vi "ADCP_write_data_packet_to_serial_port.vi"(8 "error in (no error)":errorcluster, 9 "Frame Index":i32=-1, 10 "Frame name":string, 11 "ADCP in":refnum<class "ADCP.lvclass">) -> (0 "error out":errorcluster, 3 "ADCP out":refnum<class "ADCP.lvclass">)   [LabVIEW 2017, in "ADCP.lvclass"]
uses:
  ADCP.lvclass
  ADCP.lvclass/ADCP.ctl
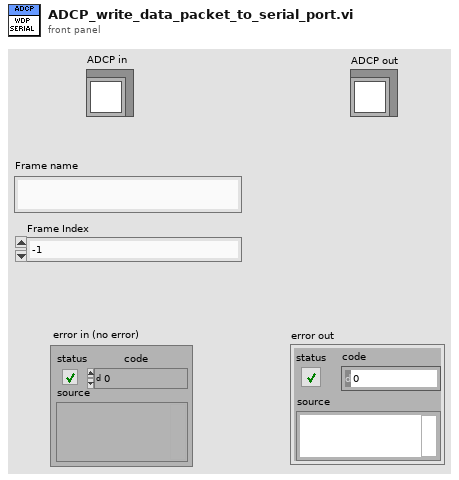
[diagram p1: front panel]
types:
  T1 = enum16{"Data", "Connection Management", "Remote Request", "Error and status", "INVALID"}
  T2 = typedef "ADCP.lvclass/ADCP_Data_Packet_Transmit_Mode.ctl" = enum16{"Disable", "Single", "Cyclic", "Repeat"}
  T3 = cluster{"Parameters":cluster{"Parameter name":string, "Node name":string, "Node ID":u8, "Frame name":string, "Frame ID":u8, "Start bit":u32, "Bit length":u32, "Factor":dbl, "Offset":dbl, "Minimum":dbl, "Maximum":dbl, "Value":string, "Comments":string, "Data_Type":enum16{"BOOL", "UNSIGNED", "SIGNED", "FLOAT32", "ENUM"}, "Enum List":string[]}[], "Priority":enum16{"LOW", "HIGH"}, "Node name":string, "Node ID":u8, "Frame name":string, "Frame ID":u8, "Data":u32, "Raw bytes":u8[], "Processed bytes":u8[], "Tx count":i32, "Last Tx Time":u32, "Tx interval":u32, "Rx count":i32, "Last Rx Time":u32, "Rx interval":u32, "Tx Enable":bool, "Tx mode":T2, "Repeat/Cyclic Tx interval":u32, "Repeat count":u16}
  T4 = cluster{"Parameters":cluster{"Parameter name":string, "Node name":string, "Node ID":u8, "Frame name":string, "Frame ID":u8, "Start bit":u32, "Bit length":u32, "Factor":dbl, "Offset":dbl, "Minimum":dbl, "Maximum":dbl, "Value":string, "Comments":string, "Data_Type":enum16{"BOOL", "UNSIGNED", "SIGNED", "FLOAT32", "ENUM"}, "Enum List":string[]}[], "Priority":enum16{"LOW", "HIGH"}, "Node name":string, "Node ID":u8, "Frame name":string, "Frame ID":u8, "Data":u32, "Raw bytes":u8[], "Processed bytes":u8[], "Tx count":i32, "Last Tx Time":u32, "Tx interval":u32, "Rx count":i32, "Last Rx Time":u32, "Rx interval":u32, "Tx Enable":bool, "Tx mode":T2, "Repeat/Cyclic Tx interval":u32, "Repeat count":u16}[]
  T5 = typedef "ADCP.lvclass/ADCP_Packet_Info.ctl" = cluster{"Priority":enum16{"LOW", "HIGH"}, "Type":enum16{"Data", "Connection Management", "Remote Request", "Error and status", "INVALID"}, "Node ID":i32, "Frame ID":i32, "Checksum valid ?":bool, "Current time (ms)":u32}
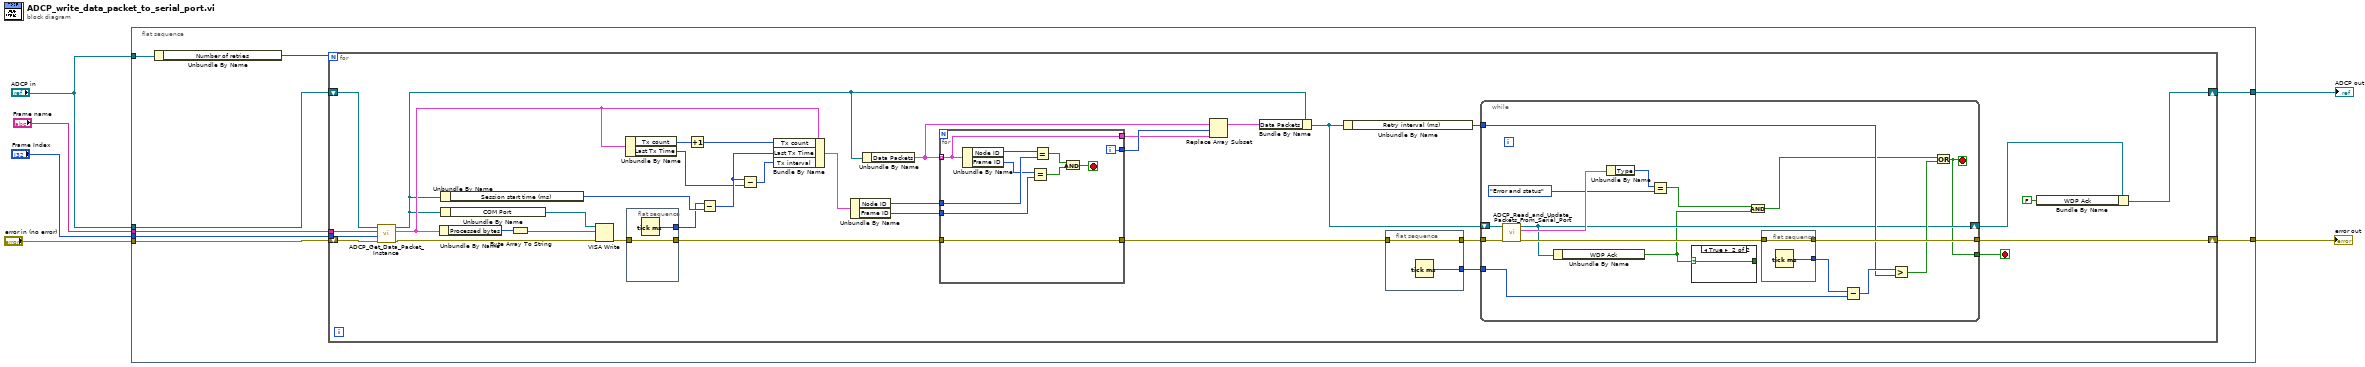
[diagram p0: block diagram]
diagram:
  n1 = flat-sequence {
    tunnel: "ADCP in" -> [w14]
    tunnel: "Frame name" -> [w13]
    tunnel: "Frame Index" -> [w12]
    tunnel: "error in (no error)" -> [w11]
    tunnel: [w10] -> w3
    tunnel: [w9] -> w2
    tunnel: "ADCP in" -> [w8]
    frame #0 {
      n2 = Unbundle By Name(w8) -> ("Number of retries"=w7:u16)
      n3 = for {
        N: w7 -> [_]
        tunnel: w13 -> [w49]
        tunnel: w12 -> [w48]
        shift-right: [w17] -> w10
        shift-left: w14 -> [w50]
        shift-right: [w16] -> w9
        shift-left: w11 -> [w47]
        stop <- w15 stop-if-true
        n4 = call "ADCP_Get_Data_Packet_Instance.vi"("error in (no error)"=w47, "Frame Index"=w48, "Frame name"=w49, "ADCP in"=w50) -> ("error out"=w46:errorcluster, "Data Packet"=w40:T3, "ADCP out"=w25:refnum<class "ADCP.lvclass">)  [unwired: 5 in]
        n5 = Unbundle By Name(w40) -> ("Processed bytes"=w44:u8[])
        n6 = Unbundle By Name(w25) -> ("Session start time (ms)"=w38:u32)
        n7 = Unbundle By Name(w25) -> ("COM Port"=w45:refnum<visa-resource-name>)
        n8 = Byte Array To String(unsigned byte array=w44) -> (string=w43:string)
        n9 = VISA Write(VISA resource name=w45, write buffer=w43, error in (no error)=w46) -> (error out=w39:errorcluster)  [unwired: 2 out]
        n10 = Unbundle By Name(w40) -> ("Tx count"=w42:i32, "Last Tx Time"=w35:u32)
        n11 = flat-sequence {
          tunnel: w39 -> [w85]
          tunnel: [w85] -> w32
          tunnel: [w84] -> w37
          frame #0 {
            n12 = Tick Count (ms)() -> (millisecond timer value=w84:u32)
          }
        }
        n13 = Increment(x=w42) -> (x+1=w41:i32)
        n14 = Subtract(x=w37, y=w38) -> (x-y=w36:u32)
        n15 = Subtract(x=w36, y=w35) -> (x-y=w34:u32)
        n16 = Bundle By Name(cluster=w40, "Tx count"=w41, "Last Tx Time"=w36, "Tx interval"=w34) -> (w33:T3)
        n17 = Unbundle By Name(w33) -> ("Node ID"=w31:u8, "Frame ID"=w30:u8)
        n18 = Unbundle By Name(w25) -> ("Data Packets"=w29:T4)
        n19 = for {
          tunnel: w32 -> [w83]
          tunnel: w31 -> [w81]
          tunnel: w30 -> [w79]
          tunnel: [w83] -> w24
          tunnel: w29 -> [w75] mode=indexing
          tunnel: [w75] -> w27
          tunnel: [w74] -> w28
          i -> [w74]
          stop <- w76 stop-if-true
          n20 = Unbundle By Name(w75) -> ("Node ID"=w82:u8, "Frame ID"=w80:u8)
          n21 = Equal?(x=w80, y=w79) -> (x = y?=w77:bool)
          n22 = Equal?(x=w82, y=w81) -> (x = y?=w78:bool)
          n23 = And(x=w78, y=w77) -> (x .and. y?=w76:bool)
        }
        n24 = Replace Array Subset(array=w29, new element=w27, index=w28) -> (w26:T4)
        n25 = Bundle By Name(cluster=w25, "Data Packets"=w26) -> (w18:refnum<class "ADCP.lvclass">)
        n26 = Unbundle By Name(w18) -> ("Retry interval (ms)"=w21:u16)
        n27 = flat-sequence {
          tunnel: w24 -> [w52]
          tunnel: [w52] -> w23
          tunnel: [w51] -> w22
          frame #0 {
            n28 = Tick Count (ms)() -> (millisecond timer value=w51:u32)
          }
        }
        n29 = while {
          tunnel: w23 -> [w69]
          shift-right: [w56] -> w20
          shift-left: w18 -> [w64]
          tunnel: w22 -> [w60]
          tunnel: [w62] -> w16
          tunnel: w21 -> [w58]
          tunnel: [w53] -> w15
          stop <- w53 stop-if-true
          n30 = call "ADCP_Read_and_Update_Packets_From_Serial_Port.vi"("error in (no error)"=w69, "ADCP In"=w64) -> ("error out"=w63:errorcluster, "Packet Info"=w68:T5, "ADCP out"=w56:refnum<class "ADCP.lvclass">)  [unwired: 6 in, 1 out]
          n31 = Unbundle By Name(w56) -> ("WDP Ack"=w55:bool)
          n32 = Unbundle By Name(w68) -> ("Type"=w67:T1)
          n33 = Equal?(x=w67, y=T1."Error and status") -> (x = y?=w65:bool)
          n34 = case shown="True" w55 {
            selector: w55 -> [w70 w71]
            tunnel: [w70 w71] -> _
            frame False {
            }
            frame True {
            }
          }
          n35 = And(x=w65, y=w55) -> (x .and. y?=w54:bool)
          n36 = flat-sequence {
            tunnel: w63 -> [w73]
            tunnel: [w73] -> w62
            tunnel: [w72] -> w61
            frame #0 {
              n37 = Tick Count (ms)() -> (millisecond timer value=w72:u32)
            }
          }
          n38 = Subtract(x=w61, y=w60) -> (x-y=w59:u32)
          n39 = Greater?(x=w59, y=w58) -> (0:w57:bool)
          n40 = Or(x=w54, y=w57) -> (x .or. y?=w53:bool)
        }
        n41 = Bundle By Name(cluster=w20, "WDP Ack"=FALSE ("Error and Status.WDP Ack")) -> (w17:refnum<class "ADCP.lvclass">)
      }
    }
  }
  "error out" <- w2
  "ADCP out" <- w3
